vi "bmp085_get_ut.vi"(8 "error in (no error)":errorcluster, 11 "BMP085 (GY-65) in":refnum<class "BMP085 (GY-65).lvclass">) -> (0 "error out":errorcluster, 2 "UT":i32, 3 "BMP085 (GY-65) out":refnum<class "BMP085 (GY-65).lvclass">)   [LabVIEW 2015, in "BMP085 (RT).lvlib" / "BMP085 (GY-65).lvclass"]
uses:
  BMP085 (GY-65).lvclass
  BMP085 (GY-65).lvclass/BMP085 (GY-65).ctl
  <vilib>/Utility/error.llb/Error Cluster From Error Code.vi
  <vilib>/myRIO/Common/Instrument Driver Framework/myRIO v1.0/I2C/vis/myRIO v1.0 Write I2C.vi
  <vilib>/myRIO/Common/Instrument Driver Framework/myRIO v1.0/I2C/vis/myRIO v1.0 Read I2C.vi
  <vilib>/myRIO/Instrument Drivers/Onboard IO/I2C/I2C.lvlib
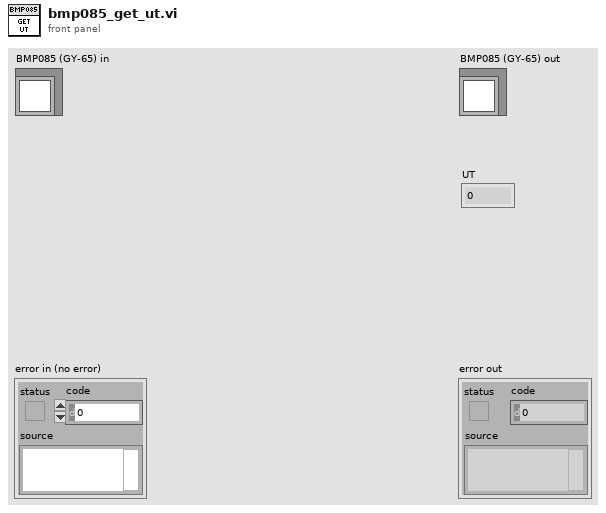
[diagram p1: front panel]
types:
  T1 = typedef "I2C.lvlib/I2C Reference.ctl" = cluster{"myRIO Reference":T2, "I2C Channels Enum":T6, "I2C Configuration":T7}
  T2 = typedef "myRIO Generic Hardware Reference.ctl" = cluster{"myRIO Model":T3, "myRIO Hardware Reference":T4}
  T3 = typedef "Hardware Version Enum.ctl" = enum16{"Unknown", "myRIO-1900", "myRIO-1950", "roboRIO"}
  T4 = typedef "myRIO v1.0 Reference.ctl" = cluster{"Generic FPGA Reference":T5, "Allow multiple opens":bool}
  T5 = typedef "Generic FPGA Reference.ctl" = refnum<k20>
  T6 = typedef "I2C Channels Enum.ctl" = enum16{"Not Connected", "A/I2C", "B/I2C", "I2C/I2C"}
  T7 = typedef "I2C.lvlib/I2C Configuration.ctl" = cluster{"I2C Transfer Rate":T8}
  T8 = typedef "I2C.lvlib/I2C Transfer Rate.ctl" = enum16{"Standard mode (100 kbps)", "Fast mode (400 kbps)"}
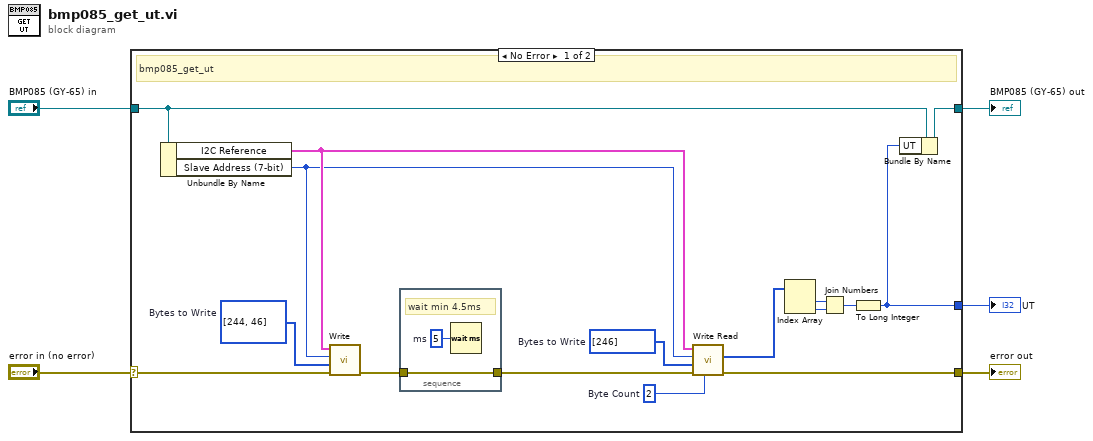
[diagram p0: block diagram]
diagram:
  n1 = case shown="No Error" "error in (no error)" {
    selector: "error in (no error)" -> [w20 w25]
    tunnel: [w8 w25] -> w4
    tunnel: [w9 w24] -> w2
    tunnel: "BMP085 (GY-65) in" -> [w21 w24]
    tunnel: [w7 _] -> w1
    frame No Error {
      w17 = u8[] [246]  # Bytes to Write
      w16 = u32 2  # Byte Count
      w19 = u8[] [244, 46]  # Bytes to Write
      # "bmp085_get_ut"
      n2 = Unbundle By Name(w21) -> ("I2C Reference"=w14:T1, "Slave Address (7-bit)"=w6:u8)
      n3 = call <vilib>:"Write.vi"("error in (no error)"=w20, "Bytes to Write"=w19, "Slave Address (7-bit)"=w6, "I2C Ref In"=w14) -> ("error out"=w18:errorcluster)  [unwired: 6 in, 1 out]
      n4 = stacked-sequence {
        tunnel: w18 -> [w22]
        tunnel: [w22] -> w15
        frame #0 {
          w23 = u32 5  # ms
          # "wait min 4.5ms"
          n5 = Wait (ms)(milliseconds to wait=w23) -> ()  [unwired: 1 out]
        }
      }
      n6 = call <vilib>:"Write Read.vi"("Byte Count"=w16, "error in (no error)"=w15, "Bytes to Write"=w17, "Slave Address (7-bit)"=w6, "I2C Ref In"=w14) -> ("error out"=w8:errorcluster, "Bytes Read"=w10:u8[])  [unwired: 3 in, 1 out]
      n7 = Index Array(array=w10) -> (element #1=w13:u8, element #2=w12:u8)  [unwired: 2 in]
      n8 = Join Numbers(hi=w13, lo=w12) -> ((hi.lo)=w11:u16)
      n9 = To Long Integer(number=w11) -> (32bit integer=w7:i32)
      n10 = Bundle By Name(cluster=w21, "UT"=w7) -> (w9:refnum<class "BMP085 (GY-65).lvclass">)
    }
    frame Error {
    }
  }
  "error out" <- w4
  "BMP085 (GY-65) out" <- w2
  "UT" <- w1
